vi "Create Query String.vi"(6 "Max Results (-1 is ALL)":i32=-1, 8 "error in (no error)":errorcluster, 9 "DataFinder parameters":T2[](array[typedef]), 10 "Return Type (ChannelGroup)":T1=enum."eSearchChannelGroup") -> (0 "error out":errorcluster, 3 "Query String Out":string)   [LabVIEW 2011]
uses:
  Datafinder Query.ctl
  eSearch Types.ctl
  DataFinder Comparisons.ctl
panel:
  out "Size":i32
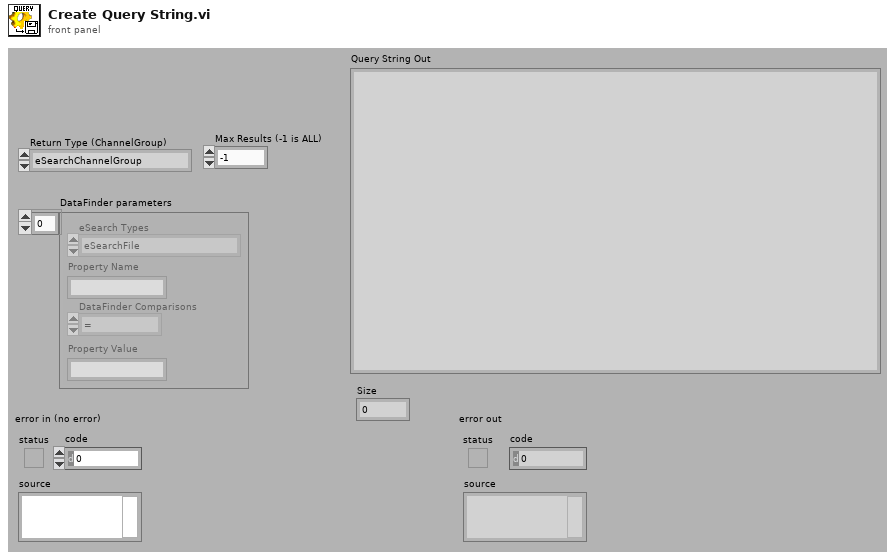
[diagram p1: front panel]
types:
  T1 = typedef "eSearch Types.ctl" = enum16{"eSearchFile", "eSearchChannelGroup", "eSearchChannel"}
  T2 = typedef "Datafinder Query.ctl" = cluster{"eSearch Types":T1, "Property Name":string, "DataFinder Comparisons":T3, "Property Value":string}
  T3 = typedef "DataFinder Comparisons.ctl" = enum16{"=", "<>", "<", "<=", ">", ">="}
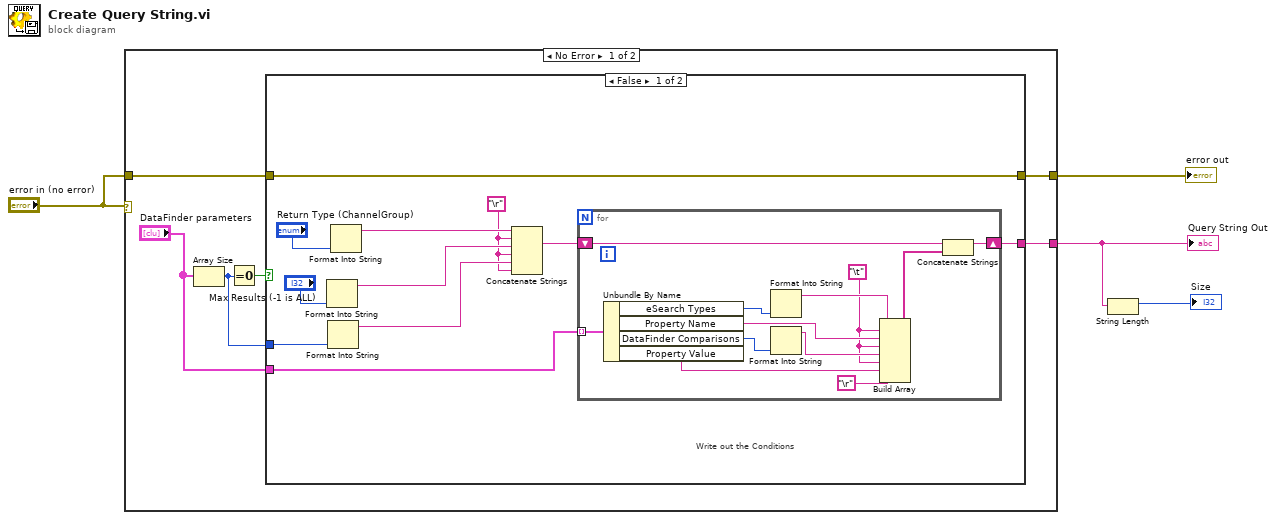
[diagram p0: block diagram]
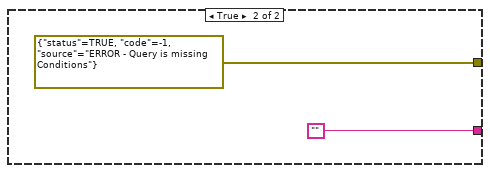
[diagram p2: hidden frame]
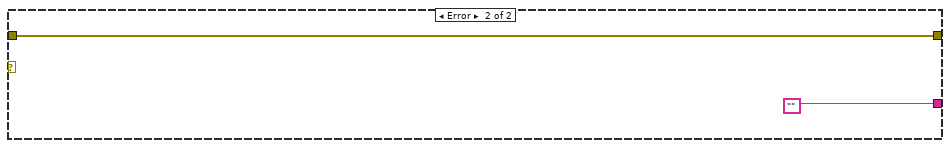
[diagram p3: hidden frame]
diagram:
  n1 = case shown="No Error" "error in (no error)" {
    tunnel: "error in (no error)" -> [w5 w37]
    tunnel: [w10 w37] -> w3
    tunnel: [w6 ""] -> w2
    frame No Error {
      n2 = Array Size(array="DataFinder parameters") -> (size(s)=w7:i32)
      n3 = Equal To 0?(x=w7) -> (x = 0?=w8:bool)
      n4 = case shown="False" w8 {
        tunnel: "DataFinder parameters" -> [w21 _]
        tunnel: [w11 errorcluster {"status"=TRUE, "code"=-1, "source"="ERROR - Query is missing Conditions"} ("error out")] -> w10
        tunnel: w7 -> [w16 _]
        tunnel: [w12 ""] -> w6
        tunnel: w5 -> [w11 _]
        frame False {
          w14 = "\r"
          # "Write out the Conditions"
          n5 = Format Into String("Max Results (-1 is ALL)") -> (resulting string=w17:string)  [unwired: 3 in, 1 out]
          n6 = Format Into String(w16) -> (resulting string=w15:string)  [unwired: 3 in, 1 out]
          n7 = Format Into String("Return Type (ChannelGroup)") -> (resulting string=w18:string)  [unwired: 3 in, 1 out]
          n8 = Concatenate Strings(w18, w14, w17, w14, w15, w14) -> (w13:string)
          n9 = for {
            tunnel: w21 -> [w33] mode=indexing
            shift-right: [w22] -> w12
            shift-left: w13 -> [w24]
            w26 = "\t"
            n10 = Unbundle By Name(w33) -> ("eSearch Types"=w32:T1, "Property Name"=w30:string, "DataFinder Comparisons"=w29:T3, "Property Value"=w27:string)
            n11 = Format Into String(w32) -> (resulting string=w31:string)  [unwired: 3 in, 1 out]
            n12 = Format Into String(w29) -> (resulting string=w28:string)  [unwired: 3 in, 1 out]
            n13 = Build Array(w31, w26, w30, w26, w28, w26, w27, "\r") -> (w23:string[])
            n14 = Concatenate Strings(w24, w23) -> (w22:string)
          }
        }
        frame True {
        }
      }
    }
    frame Error {
    }
  }
  "error out" <- w3
  "Query String Out" <- w2
  n15 = String Length(string=w2) -> (length=→"Size":i32)
